vi "Write_Html_Report_Sub_VI.vi"(1 "ReprtPath":string, 2 "Remarks":string, 3 "Iterations":i64, 4 "Error Description":string, 6 "Timestamp":string, 7 "TestCase":string, 8 "Verdict":string, 9 "TestSuite":string, 10 "Time taken to execute  test in msec":string, 11 "JazzDashboardLink":string, 12 "Delay Between Iterations":i64=1000, 13 "Error Code":i32) -> ()   [LabVIEW 2017]
uses:
  <vilib>/Utility/NIReport.llb/Append Report Text (str wrap).vi
  <vilib>/Utility/NIReport.llb/Append Text Table to Report (wrap).vi
  <vilib>/Utility/NIReport.llb/Append Image to Report (path wrap).vi
  <vilib>/Utility/NIReport.llb/NI_report.lvclass
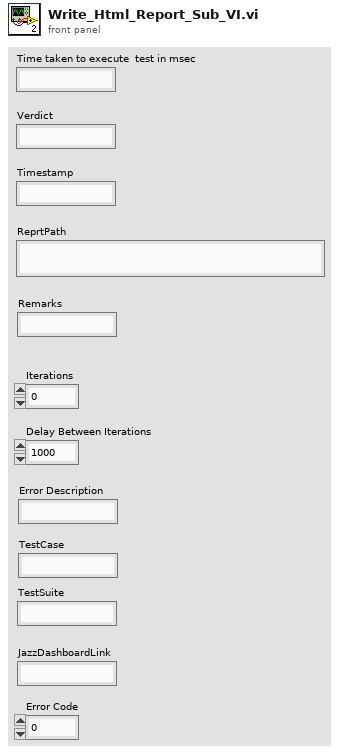
[diagram p1: front panel]
types:
  T1 = enum16{"Standard Report", "HTML", "Word", "Excel"}
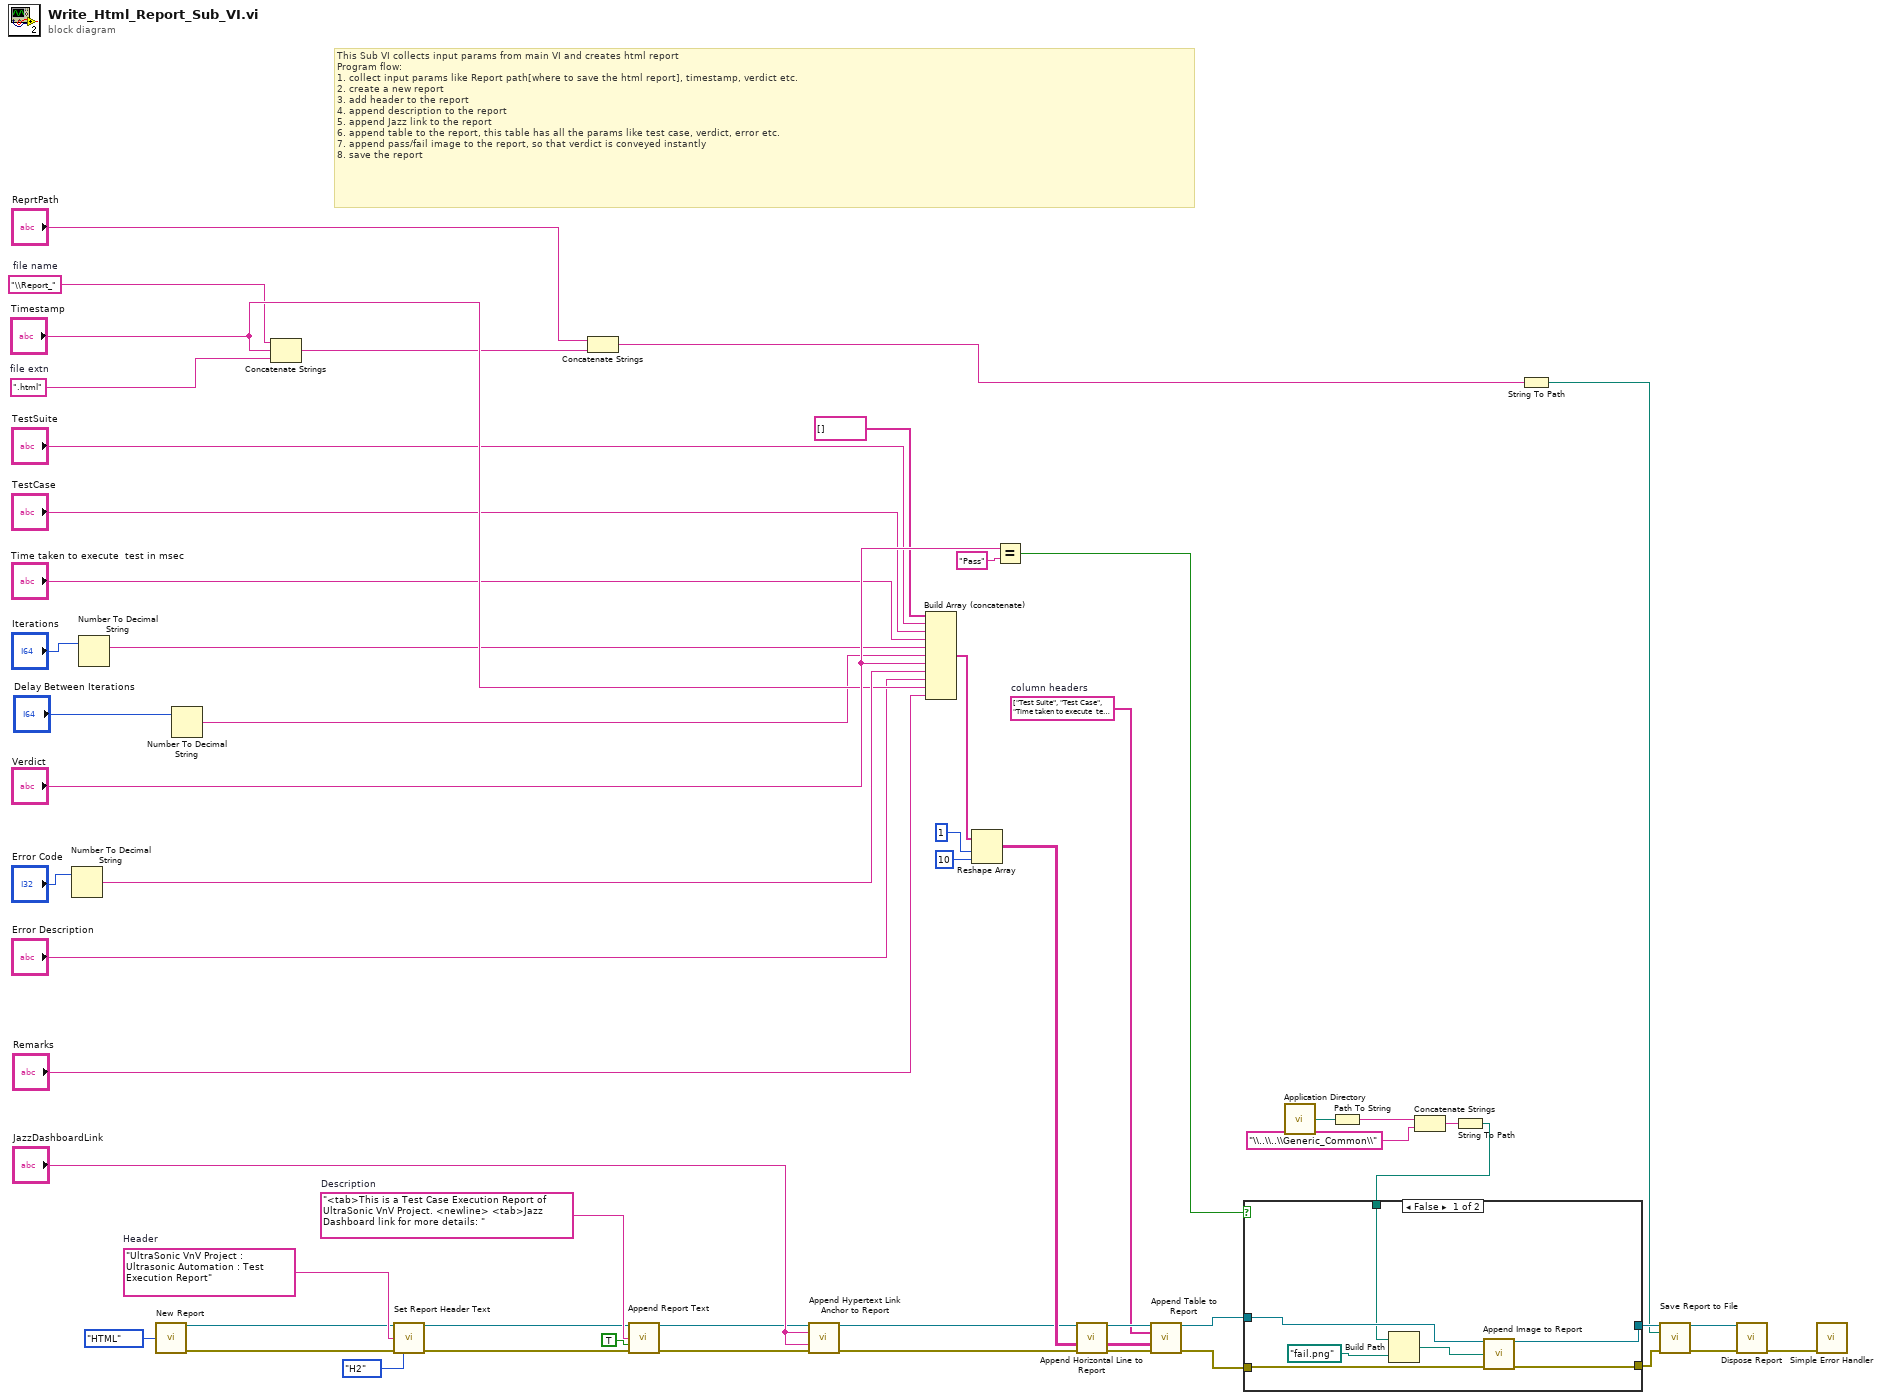
[diagram p0: block diagram]
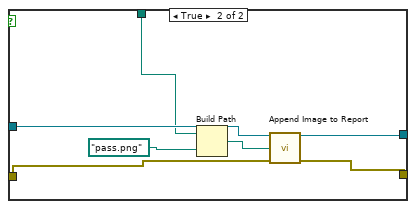
[diagram p2: hidden frame]
diagram:
  w8 = "\\Report_"  # file name
  w21 = "<tab>This is a Test Case Execution Report of UltraSonic VnV Project. <newline> <tab>Jazz Dashboard link for more details: "  # Description
  w16 = "UltraSonic VnV Project : Ultrasonic Automation : Test Execution Report"  # Header
  w40 = ".html"  # file extn
  w26 = string[] ["Test Suite", "Test Case", "Time taken to execute  test (msec)", "Number of times test executed (Iterations)", "Delay Between Iterations (msec)", "Verdict", "Error Code", "Error Description", "Timestamp", "Remarks"]  # column headers
  # "This Sub VI collects input params from main VI and creates html report\nProgram flow:\n1. collect input params like Report path[where to save the html report], timestamp, verdict etc.\n2. create a new report \n3. add header to the report\n4. append description to the report\n5. append Jazz link to the report\n6. append table to the report, this table has all the params like test case, verdict, error etc.\n7. append pass/fail image to the report, so that verdict is conveyed instantly\n8. save the report"
  n1 = Number To Decimal String(number="Error Code") -> (decimal integer string=w52:string)  [unwired: 1 in]
  n2 = Number To Decimal String(number="Iterations") -> (decimal integer string=w10:string)  [unwired: 1 in]
  n3 = call <vilib>:"New Report.vi"("report type"=T1."HTML") -> ("report out"=w15:refnum<class "NI_report.lvclass">, "error out"=w14:errorcluster)  [unwired: 13 in]
  n4 = Number To Decimal String(number="Delay Between Iterations") -> (decimal integer string=w6:string)  [unwired: 1 in]
  n5 = Concatenate Strings "Concatenate Strings"(w8, "Timestamp", w40) -> (w39:string)
  n6 = call-dynamic "Set Report Header Text.vi"("report in"=w15, "center header text"=w16, "error in (no error)"=w14, "HTML header size"=enum16{"H1", "H2", "H3", "H4", "H5", "H6", "H7"}."H2") -> ("report out"=w19:refnum<class "NI_report.lvclass">, "error out"=w23:errorcluster)  [unwired: 10 in]
  n7 = Concatenate Strings "Concatenate Strings"("ReprtPath", w39) -> (w41:string)
  n8 = call-poly <vilib>:"Append Report Text.vi"("report in"=w19, "text"=w21, "append on new line? (F)"=TRUE, "error in (no error)"=w23) -> ("report out"=w27:refnum<class "NI_report.lvclass">, "error out"=w28:errorcluster)  [unwired: 8 in, 2 out]
  n9 = call-dynamic "Append Hypertext Link Anchor to Report.vi"("report in"=w27, "URL of link - href"="JazzDashboardLink", "link text"="JazzDashboardLink", "error in (no error)"=w28) -> ("report out"=w32:refnum<class "NI_report.lvclass">, "error out"=w31:errorcluster)  [unwired: 8 in, 2 out]
  n10 = Build Array (concatenate)(string[] [] ("array"), "TestSuite", "TestCase", "Time taken to execute  test in msec", w10, w6, "Verdict", w52, "Error Description", "Timestamp", "Remarks") -> (w34:string[])
  n11 = Reshape Array "Reshape Array"(w34, 1 ("dimension size"), 10 ("dimension size")) -> (w37:string[][])
  n12 = Equal?(x="Verdict", y="Pass") -> (x = y?=w48:bool)
  n13 = call-dynamic "Append Horizontal Line to Report.vi"("report in"=w32, "error in (no error)"=w31) -> ("report out"=w29:refnum<class "NI_report.lvclass">, "error out"=w30:errorcluster)  [unwired: 12 in]
  n14 = call-poly <vilib>:"Append Table to Report.vi"("report in"=w29, "column headers"=w26, "text data"=w37, "error in (no error)"=w30) -> ("report out"=w43:refnum<class "NI_report.lvclass">, "error out"=w46:errorcluster)  [unwired: 8 in, 2 out]
  n15 = call <vilib>:"Application Directory.vi"() -> ("Application Directory"=w2:path)
  n16 = Path To String(path=w2) -> (string=w4:string)
  n17 = Concatenate Strings(w4, "\\..\\..\\Generic_Common\\" ("string")) -> (w5:string)
  n18 = String To Path(string=w5) -> (path=w1:path)
  n19 = case shown="False" w48 {
    tunnel: w43 -> [w62 w69]
    tunnel: [w59 w68] -> w44
    tunnel: [w60 w67] -> w45
    tunnel: w46 -> [w61 w66]
    tunnel: w1 -> [w56 w63]
    frame False {
      n20 = Build Path(base path=w56, name or relative path=path "fail.png" ("default name")) -> (appended path=w57:path)
      n21 = call-poly <vilib>:"Append Image to Report.vi"("report in"=w62, "path or URL of image"=w57, "error in (no error)"=w61) -> ("report out"=w59:refnum<class "NI_report.lvclass">, "error out"=w60:errorcluster)  [unwired: 9 in, 2 out]
    }
    frame True {
      n22 = Build Path(base path=w63, name or relative path=path "pass.png" ("default name")) -> (appended path=w64:path)
      n23 = call-poly <vilib>:"Append Image to Report.vi"("report in"=w69, "path or URL of image"=w64, "error in (no error)"=w66) -> ("report out"=w68:refnum<class "NI_report.lvclass">, "error out"=w67:errorcluster)  [unwired: 9 in, 2 out]
    }
  }
  n24 = String To Path(string=w41) -> (path=w38:path)
  n25 = call-dynamic "Save Report to File.vi"("report in"=w44, "report file path"=w38, "error in (no error)"=w45) -> ("report out"=w25:refnum<class "NI_report.lvclass">, "error out"=w24:errorcluster)  [unwired: 11 in]
  n26 = call-dynamic "Dispose Report.vi"("report in"=w25, "error in (no error)"=w24) -> ("error out"=w20:errorcluster)  [unwired: 13 in]
  n27 = call <vilib>:"Simple Error Handler.vi"("error in (no error)"=w20) -> ()  [unwired: 4 in, 5 out]
